vi "AutoDriveStraightWeird.vi"(8 "error in (no error)":errorcluster, 9 "TimeOut (s)":dbl, 10 "MaxSpeed (ft/s)":dbl, 11 "Dist (ft)":dbl) -> (0 "error out":errorcluster)   [LabVIEW 2020]
doc: "Wrapper class for drive straight"
uses:
  <vilib>/Rock Robotics/WPI/ThirdParty/JAS_Junk/TrajLib/Trajectory_Library.lvlib
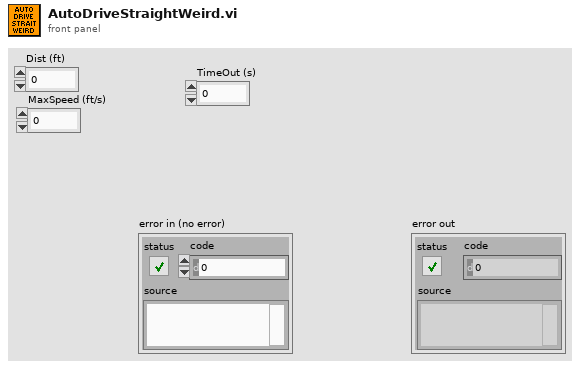
[diagram p1: front panel]
types:
  T1 = typedef "Trajectory_Library.lvlib/TIMER.ctl" = cluster{"StartTime":dbl, "Accumulated TIme":dbl, "Running":bool, "semaphore":T2}
  T2 = typedef "Semaphore RefNum" = refnum<k1>
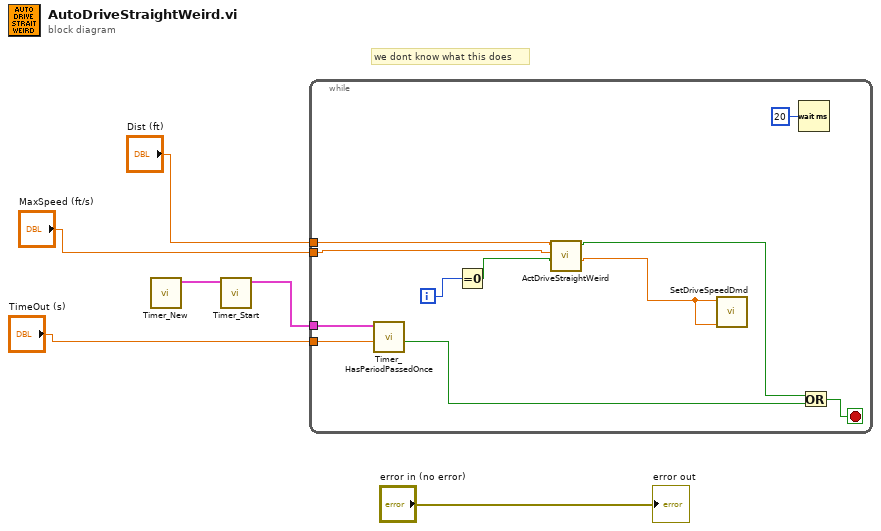
[diagram p0: block diagram]
diagram:
  # "we dont know what this does"
  n1 = call <vilib>:"Timer_New.vi"() -> ("TIMER"=w3:T1)  [unwired: 11 in]
  n2 = call <vilib>:"Timer_Start.vi"("in Timer"=w3) -> ("out Timer"=w2:T1)  [unwired: 10 in]
  n3 = while {
    tunnel: "Dist (ft)" -> [w8]
    tunnel: "MaxSpeed (ft/s)" -> [w9]
    tunnel: w2 -> [w16]
    tunnel: "TimeOut (s)" -> [w15]
    i -> [w17]
    stop <- w13 stop-if-true
    n4 = call <vilib>:"Timer_HasPeriodPassedOnce.vi"("Period"=w15, "in Timer"=w16) -> ("Expired"=w14:bool)  [unwired: 7 in, 2 out]
    n5 = Equal To 0?(x=w17) -> (x = 0?=w10:bool)
    n6 = call "ActDriveStraightWeird.vi"("FirstTime"=w10, "MaxSpeed (ft/s)"=w9, "Dist (ft)"=w8) -> ("XSpeedDemand"=w7:dbl, "Done"=w11:bool)  [unwired: 7 in]
    n7 = call "SetDriveSpeedDmd.vi"("LeftSpeedInput"=w7, "RightSpeedInput"=w7) -> ()  [unwired: 10 in]
    n8 = Wait (ms)(milliseconds to wait=u32 20) -> ()  [unwired: 1 out]
    n9 = Or(x=w11, y=w14) -> (x .or. y?=w13:bool)
  }
  "error out" <- "error in (no error)"
